vi "eFGV - Sequence Data.vi"(6 "States":T2, 8 "Error In":errorcluster, 10 "Sequence Data":T1[](array[typedef])) -> (0 "Error Out":errorcluster, 2 "Event - Sequence Data":refnum<user-event>, 3 "Sequence Data Out":T1[](array[typedef]))   [LabVIEW 2020]
uses:
  Control/State - eFGV.ctl
  Control/Setup - Sequence Data.ctl
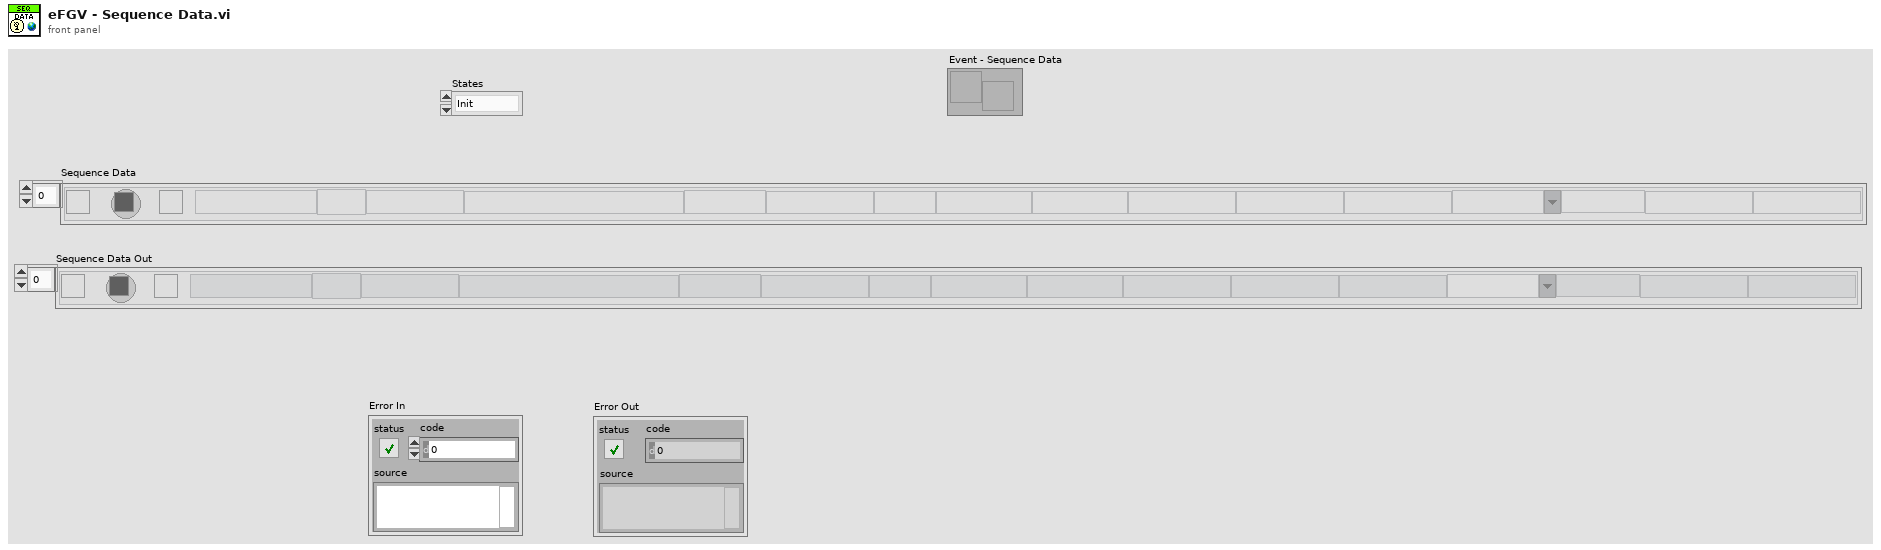
[diagram p1: front panel]
types:
  T1 = typedef "Setup - Sequence Data.ctl" = cluster{"Seq.Select":bool, "Seq.Status":u32, "Seq.Run":bool, "Seq.TestSequence":string, "Seq.No":string, "Seq.ReqID":string, "Seq.TestReq":string, "Seq.Variance":string, "Seq.TestProcedure":string, "Seq.Section":string, "Seq.TestBunker":string, "Seq.TestMedia":string, "Seq.TestPressure":string, "Seq.Cycle":string, "Seq.HoldingTime":string, "Seq.ChartScale":string, "Seq.BDIndicator":string, "Seq.ActuatorPressure":string, "Seq.MaxBDPressure":string}
  T2 = typedef "State - eFGV.ctl" = enum16{"Init", "Read", "Write", "Exit"}
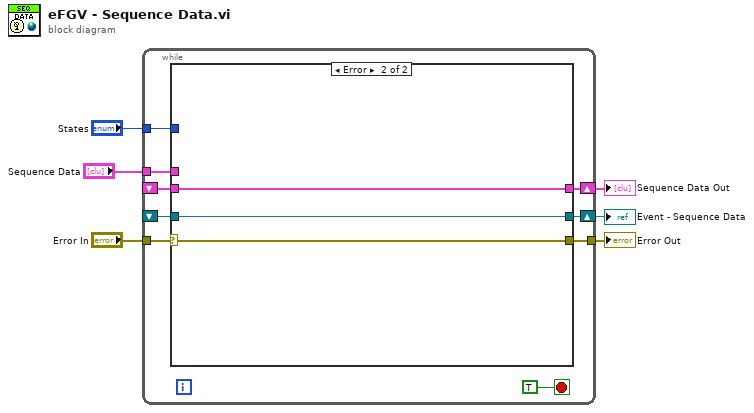
[diagram p0: block diagram]
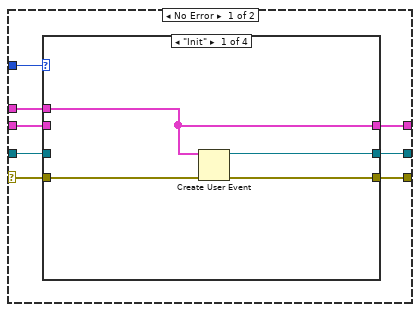
[diagram p2: hidden frame]
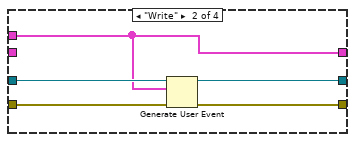
[diagram p3: hidden frame]
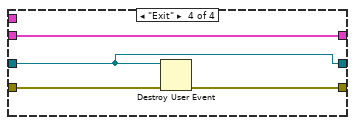
[diagram p5: hidden frame]
diagram:
  n1 = while {
    tunnel: "Error In" -> [w14]
    tunnel: [w13] -> w5
    tunnel: "States" -> [w12]
    tunnel: "Sequence Data" -> [w11]
    shift-right: [w10] -> w2
    shift-left: _ -> [w7]
    shift-right: [w9] -> w1
    shift-left: _ -> [w8]
    stop <- TRUE stop-if-true
    n2 = case shown="Error" w14 {
      selector: w14 -> [w22 w42]
      tunnel: [w21 w42] -> w13
      tunnel: w12 -> [w23 _]
      tunnel: w11 -> [w20 _]
      tunnel: [w19 w41] -> w10
      tunnel: [w18 w40] -> w9
      tunnel: w8 -> [w17 w40]
      tunnel: w7 -> [w16 w41]
      frame No Error {
        n3 = case shown="\"Init\"" w23 {
          tunnel: w22 -> [w27 w32 w35 w39]
          tunnel: [w26 w31 w35 w38] -> w21
          tunnel: w20 -> [w24 w29 _ _]
          tunnel: [w24 w29 w33 w36] -> w19
          tunnel: [w25 w28 w34 w37] -> w18
          tunnel: w17 -> [_ w30 w34 w37]
          tunnel: w16 -> [_ _ w33 w36]
          frame "Init" {
            n4 = Create User Event(user event datatype=w24, error in=w27) -> (user event=w25:refnum<user-event>, error out=w26:errorcluster)
          }
          frame "Write" {
            n5 = Generate User Event(user event=w30, event data cluster=w29, error in=w32) -> (user event out=w28:refnum<user-event>, error out=w31:errorcluster)  [unwired: 1 in]
          }
          frame "Read" {
          }
          frame "Exit" {
            n6 = Destroy User Event(user event=w37, error in=w39) -> (error out=w38:errorcluster)
          }
        }
      }
      frame Error {
      }
    }
  }
  "Error Out" <- w5
  "Sequence Data Out" <- w2
  "Event - Sequence Data" <- w1
